vi "Text to UTF-8 (LabVIEW String).vi"(8 "error in":errorcluster, 10 "Encoding (system default=-1)":i32=-1, 11 "String":string) -> (0 "error out":errorcluster, 3 "UTF-8 Encoded String":T1)   [LabVIEW 2020, in "G-Unicode.lvlib"]
uses:
  G-Unicode.lvlib
  Types/Encoded UTF-8 String.ctl
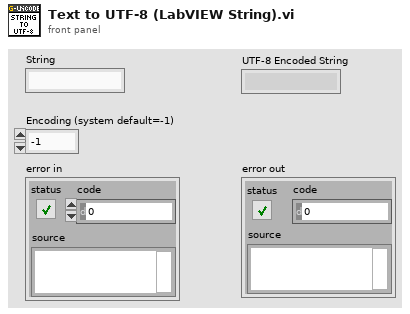
[diagram p1: front panel]
types:
  T1 = typedef "G-Unicode.lvlib/Encoded UTF-8 String.ctl" = string
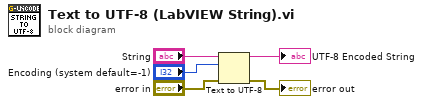
[diagram p0: block diagram]
diagram:
  n1 = Text to UTF-8(8:"error in", 10:"Encoding (system default=-1)", 11:"String") -> (0:→"error out":errorcluster, 3:→"UTF-8 Encoded String":string)
